vi "FPGA_DIOReadDO.vi"(8 "error in (no error)":errorcluster, 11 "DIODeviceRef In":T1) -> (0 "error out":errorcluster, 2 "DO":u32, 3 "DIODeviceRef Out":T1)   [LabVIEW 2017]
uses:
  <vilib>/Rock Robotics/SystemInterfaces/DIO/FPGA_DIODevRef.ctl
  <vilib>/Rock Robotics/SystemInterfaces/System/FPGA_SystemFPGA Ref Global.vi
  <vilib>/Utility/error.llb/Error Cluster From Error Code.vi
  <vilib>/rvi/errors/niLvFpgaAdjustHostInterfaceError.vi
  <vilib>/rvi/interface/nirviReadWriteControl/nirviReadWriteControl.xnode
  <vilib>/Rock Robotics/SystemInterfaces/System/FPGA_SystemFRC FPGA Ref.ctl
  NiFpgaLv.dll
  <vilib>/rvi/interface/Simulation/niFpgaSimulationCallBeginRW.vi
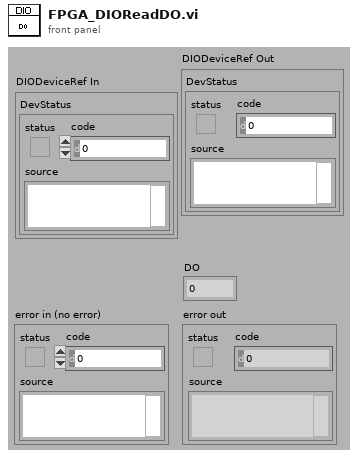
[diagram p1: front panel]
types:
  T1 = typedef "FPGA_DIODevRef.ctl" = cluster{"DevStatus":errorcluster}
  T2 = typedef "FPGA_SystemFRC FPGA Ref.ctl" = refnum<k20>
  T3 = cluster{"Headers":fxp<+,10,10>, "SPIPort":fxp<+,5,5>, "Reserved":fxp<+,1,1>, "MXP":u16}
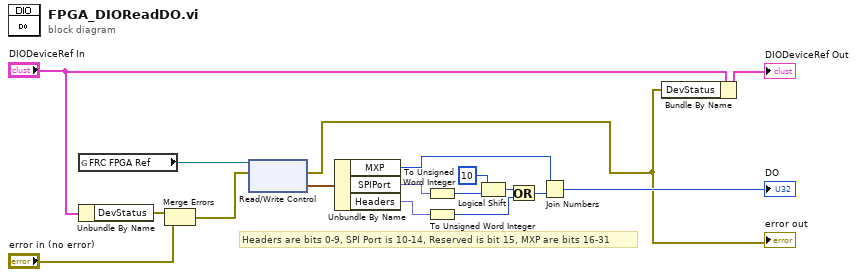
[diagram p0: block diagram]
diagram:
  # "Headers are bits 0-9, SPI Port is 10-14, Reserved is bit 15, MXP are bits 16-31"
  n1 = global read "FPGA_SystemFPGA Ref Global.vi" "FRC FPGA Ref"() -> (w14:T2)
  n2 = Unbundle By Name("DIODeviceRef In") -> ("DevStatus"=w13:errorcluster)
  n3 = Merge Errors(w13, "error in (no error)") -> (w12:errorcluster)
  n4 = xnode "Read/Write Control"("FPGA VI Reference In"=w14, "error in"=w12) -> ("error out"=w15:errorcluster, "DIO.DO"=w1:T3)  [unwired: 1 out]
  "error out" <- w15
  n5 = Unbundle By Name(w1) -> ("MXP"=w9:u16, "SPIPort"=w2:fxp<+,5,5>, "Headers"=w7:fxp<+,10,10>)
  n6 = To Unsigned Word Integer(number=w2) -> (unsigned 16bit integer=w4:u16)
  n7 = To Unsigned Word Integer(number=w7) -> (unsigned 16bit integer=w8:u16)
  n8 = Logical Shift(y=i16 10, x=w4) -> (x << y=w6:u16)
  n9 = Or(x=w6, y=w8) -> (x .or. y?=w5:u16)
  n10 = Join Numbers(hi=w9, lo=w5) -> ((hi.lo)=→"DO":u32)
  n11 = Bundle By Name(cluster="DIODeviceRef In", "DevStatus"=w15) -> (→"DIODeviceRef Out":T1)
